vi "exercise3b.vi"() -> ()   [LabVIEW 2010]
panel:
  out "i1 >= i2":bool
  in  "Input 2":dbl
  in  "Input 1":dbl
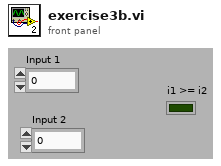
[diagram p1: front panel]
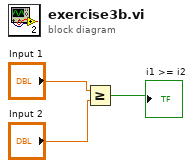
[diagram p0: block diagram]
diagram:
  n1 = Greater Or Equal?(x="Input 1", y="Input 2") -> (x >= y?=→"i1 >= i2":bool)
